vi "Join 10 To 20.vi"(2 "IN 19:10":fxp<+,10,10> format="%08b", 3 "IN 9:0":fxp<+,10,10> format="%08b") -> (1 "OUT 19:0":fxp<+,20,20> format="%08b")   [LabVIEW 2019]
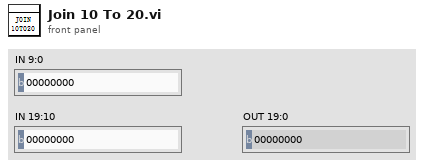
[diagram p1: front panel]
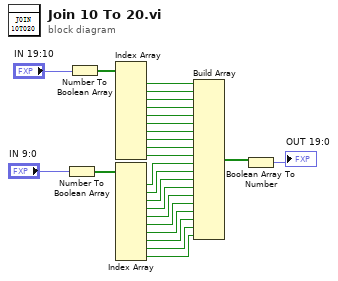
[diagram p0: block diagram]
diagram:
  n1 = Number To Boolean Array(number="IN 9:0") -> (Boolean array=w23:bool[])
  n2 = Number To Boolean Array(number="IN 19:10") -> (Boolean array=w24:bool[])
  n3 = Index Array(array=w24) -> (element #1=w22:bool, element #2=w21:bool, element #3=w20:bool, element #4=w19:bool, element #5=w18:bool, element #6=w17:bool, element #7=w16:bool, element #8=w15:bool, element #9=w14:bool, element #10=w13:bool)  [unwired: 10 in]
  n4 = Index Array(array=w23) -> (element #1=w12:bool, element #2=w11:bool, element #3=w10:bool, element #4=w9:bool, element #5=w8:bool, element #6=w7:bool, element #7=w6:bool, element #8=w5:bool, element #9=w4:bool, element #10=w3:bool)  [unwired: 10 in]
  n5 = Build Array(w22, w21, w20, w19, w18, w17, w16, w15, w14, w13, w12, w11, w10, w9, w8, w7, w6, w5, w4, w3) -> (w2:bool[])
  n6 = Boolean Array To Number ("布尔数组至数值转换")(Boolean array=w2) -> (number=→"OUT 19:0":fxp<+,20,20>)
